vi "slit_GUI.vi"(4 "error in (no error)":errorcluster, 7 "connection ID":refnum<k5>) -> (0 "error out":errorcluster)   [LabVIEW 2015]
doc: "Use this template to build a PDA VI for Pocket PC 2002 devices or emulators."
panel:
  in  "SERVICE":bool
  out "Slit Names":string
  in  "Cancel":bool
  in  "OK":bool
  in  "Slit #":u16(ring) items=["None", "1", "2", "3", "4", "5", "6", "7", "8", "9", "10", "11", "12", "13", "14", "15", "16", "17", "18", "19", "20", "21", "22", "23", "24", "25", "26", "27", "28", "29", "30", "31", "32", "33", "34", "35", "36"]
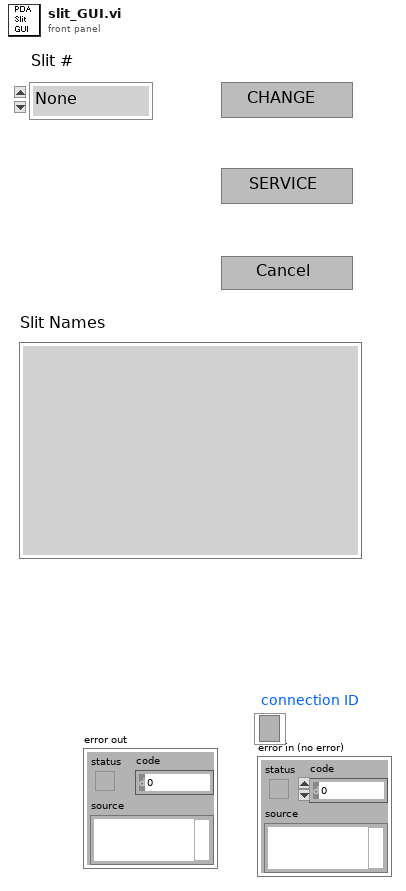
[diagram p1: front panel]
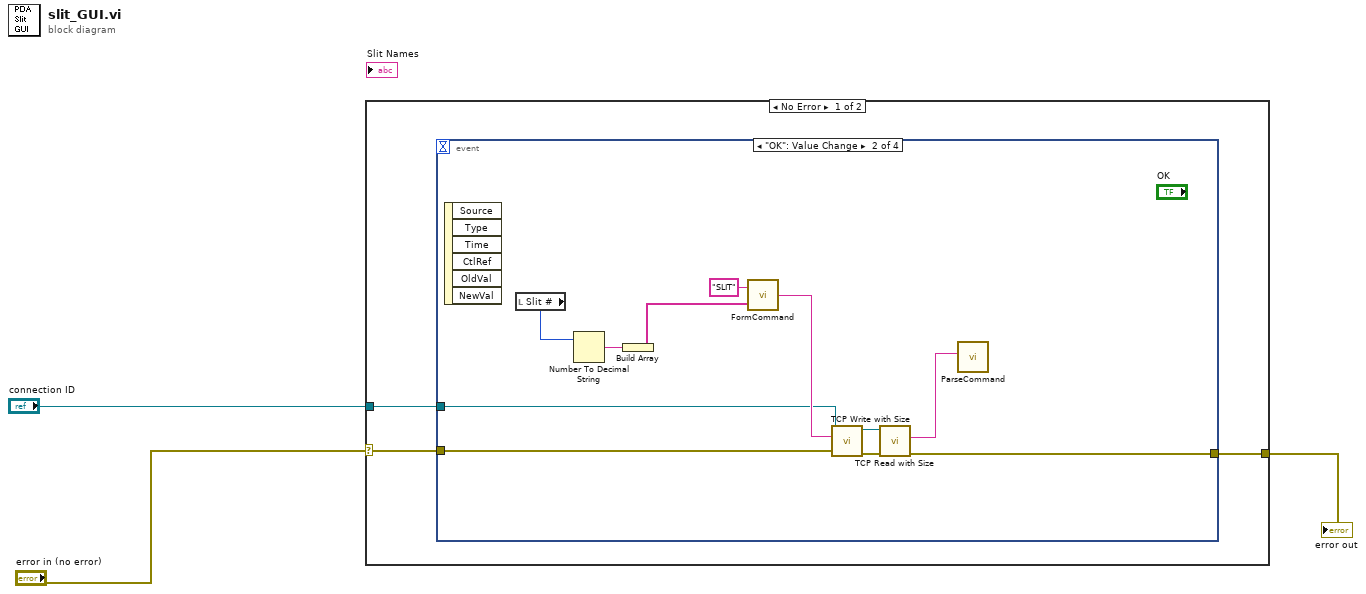
[diagram p0: block diagram]
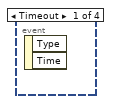
[diagram p2: hidden frame]
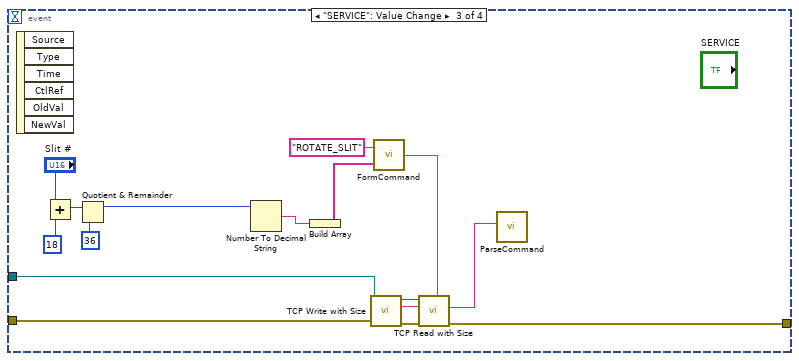
[diagram p3: hidden frame]
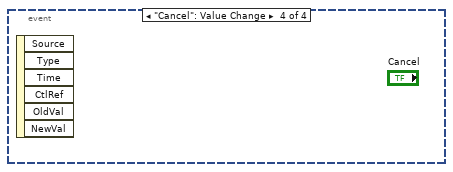
[diagram p4: hidden frame]
diagram:
  n1 = case shown="No Error" "error in (no error)" {
    selector: "error in (no error)" -> [w5 w33]
    tunnel: [w6 w33] -> w3
    tunnel: "connection ID" -> [w4 _]
    frame No Error {
      n2 = event shown="[1] \"OK\": Value Change" {
        selector: _ -> [_ _ _ _]
        dyn-events: _ -> [_ _ _ _]
        timeout: _ -> [_ _ _ _]
        tunnel: [_ w8 w20 _] -> w6
        tunnel: w5 -> [_ w9 w32 _]
        tunnel: w4 -> [_ w10 w31 _]
        event Timeout {
          n3 = event-data() -> ()  [unwired: 1 in, 2 out]
        }
        event "OK": Value Change {
          n4 = event-data() -> ()  [unwired: 1 in, 6 out]
          n5 = local read "Slit #"() -> (w7:u16)
          n6 = Number To Decimal String(number=w7) -> (decimal integer string=w16:string)  [unwired: 1 in]
          n7 = Build Array(w16) -> (w15:string[])
          n8 = call "FormCommand.vi"("Parameters"=w15, "Command"="SLIT") -> ("Command string"=w14:string)
          n9 = call "TCP Write with Size.vi"("error in (no error)"=w9, "data in"=w14, "connection ID"=w10) -> ("error out"=w13:errorcluster, "connection ID out"=w12:refnum<k5>)  [unwired: 6 in, 1 out]
          n10 = call "TCP Read with Size.vi"("error in (no error)"=w13, "connection ID"=w12) -> ("error out"=w8:errorcluster, "data out"=w11:string)  [unwired: 7 in, 1 out]
          n11 = call "ParseCommand.vi"("Command string"=w11) -> ()  [unwired: 2 out]
        }
        event "SERVICE": Value Change {
          n12 = event-data() -> ()  [unwired: 1 in, 6 out]
          n13 = Add(x="Slit #", y=18) -> (x+y=w28:i32)
          n14 = Quotient & Remainder(x=w28, y=36) -> (x-y*floor(x/y)=w19:i32)  [unwired: 1 out]
          n15 = Number To Decimal String(number=w19) -> (decimal integer string=w26:string)  [unwired: 1 in]
          n16 = Build Array(w26) -> (w25:string[])
          n17 = call "FormCommand.vi"("Parameters"=w25, "Command"="ROTATE_SLIT") -> ("Command string"=w24:string)
          n18 = call "TCP Write with Size.vi"("error in (no error)"=w32, "data in"=w24, "connection ID"=w31) -> ("error out"=w23:errorcluster, "connection ID out"=w22:refnum<k5>)  [unwired: 6 in, 1 out]
          n19 = call "TCP Read with Size.vi"("error in (no error)"=w23, "connection ID"=w22) -> ("error out"=w20:errorcluster, "data out"=w21:string)  [unwired: 7 in, 1 out]
          n20 = call "ParseCommand.vi"("Command string"=w21) -> ()  [unwired: 2 out]
        }
        event "Cancel": Value Change {
          n21 = event-data() -> ()  [unwired: 1 in, 6 out]
        }
      }
    }
    frame Error {
    }
  }
  "error out" <- w3
